vi "Test Data Trimming.vi"() -> ()   [LabVIEW 2018]
panel:
  out "time":dbl
  out "array for saving":sgl[](array[numeric])
  in  "start pixel":i32
  in  "#A-lines per B-line":i32=2048
  in  "#pixels to save":i32=200
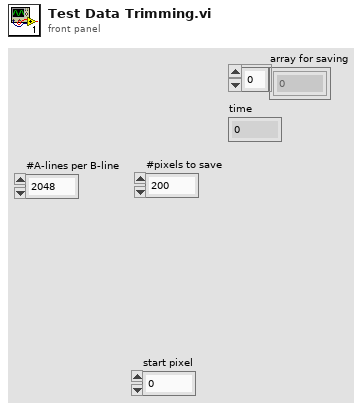
[diagram p1: front panel]
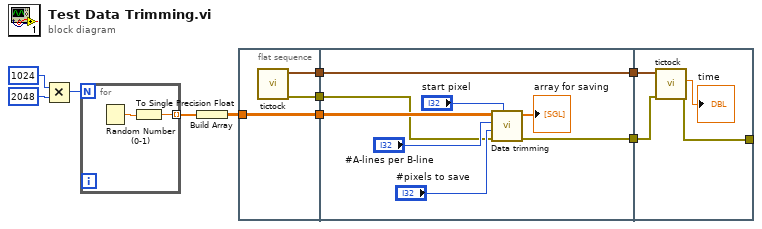
[diagram p0: block diagram]
diagram:
  n1 = Multiply(x=1024, y=2048) -> (x*y=w8:i32)
  n2 = for {
    N: w8 -> [_]
    tunnel: [w11] -> w7 mode=indexing
    n3 = Random Number (0-1)() -> (number: 0 to 1=w12:dbl)
    n4 = To Single Precision Float(number=w12) -> (single precision float=w11:sgl)
  }
  n5 = Build Array(w7) -> (w6:sgl[][])
  n6 = flat-sequence {
    tunnel: w6 -> [w15]
    tunnel: [w15] -> w5
    tunnel: [w14] -> w3
    tunnel: [w13] -> w2
    tunnel: w5 -> [w20]
    tunnel: [w18] -> w4
    tunnel: w3 -> [w18]
    tunnel: w2 -> [w17]
    tunnel: [w16] -> w1
    tunnel: w4 -> [w27]
    tunnel: w1 -> [w25]
    tunnel: [w24] -> _
    frame #0 {
      n7 = call "tictock.vi"() -> ("error out"=w13:errorcluster, "seconds since 1Jan1904"=w14:timestamp)  [unwired: 9 in, 1 out]
    }
    frame #1 {
      n8 = call "Data trimming.vi"("start pixel"="start pixel", "error in"=w17, "#pixels to save"="#pixels to save", "#A-lines"="#A-lines per B-line", "2D Array in"=w20) -> ("error out"=w16:errorcluster, "array for saving"=→"array for saving":sgl[])  [unwired: 4 in, 1 out]
    }
    frame #2 {
      n9 = call "tictock.vi"("error in (no error)"=w25, "seconds since 1Jan1904 2"=w27) -> ("error out"=w24:errorcluster, "Numeric"=→"time":dbl)  [unwired: 7 in, 1 out]
    }
  }
